vi "login3.vi"() -> ()   [LabVIEW 2023]
panel:
  in  "Tab Control":enum32{"Page 1", "Page 2"}(tab)
  in  "refresh button":bool
  in  "Username":string
  in  "Password":string
  out "LED":bool
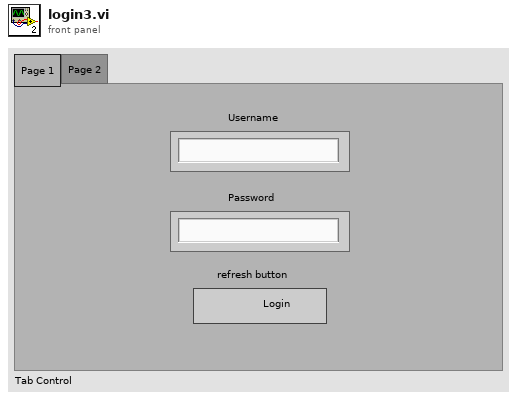
[diagram p1: front panel]
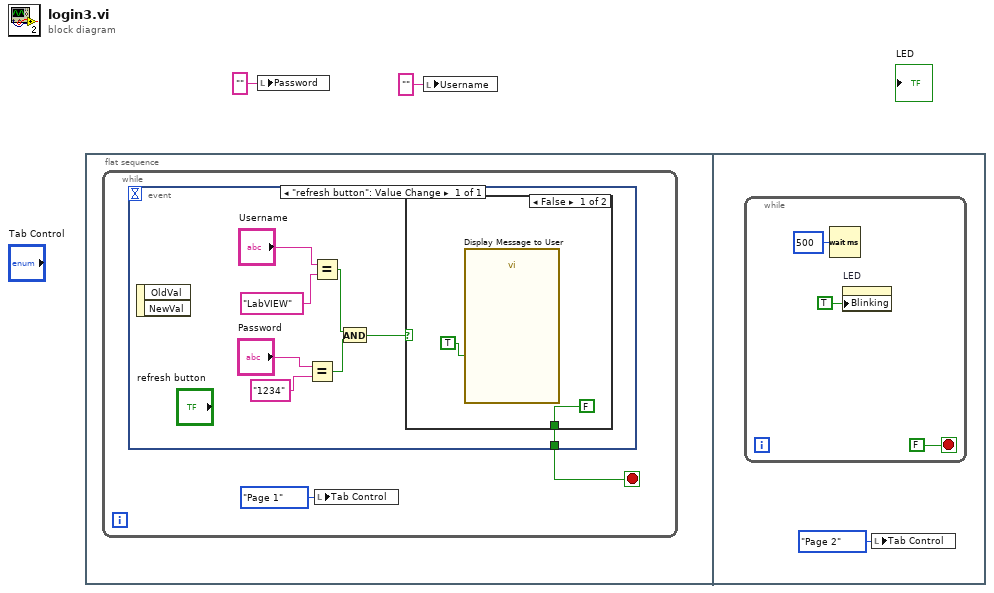
[diagram p0: block diagram]
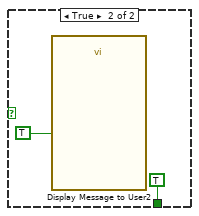
[diagram p2: hidden frame]
diagram:
  n1 = flat-sequence {
    frame #0 {
      n2 = while {
        stop <- w4 stop-if-true
        n3 = event shown="[0] \"refresh button\": Value Change" {
          selector: _ -> [_]
          dyn-events: _ -> [_]
          timeout: _ -> [_]
          tunnel: [w5] -> w4
          event "refresh button": Value Change {
            n4 = event-data() -> ()  [unwired: 1 in, 2 out]
            n5 = Equal?(x="Password", y="1234") -> (x = y?=w9:bool)
            n6 = Equal?(x="Username", y="LabVIEW") -> (x = y?=w10:bool)
            n7 = And(x=w10, y=w9) -> (x .and. y?=w8:bool)
            n8 = case shown="False" w8 {
              tunnel: [FALSE TRUE] -> w5
              frame False {
                n9 = call "Display Message to User"("Enable"=TRUE) -> ()  [unwired: 9 in, 2 out]
              }
              frame True {
                n10 = call "Display Message to User2"("Enable"=TRUE) -> ()  [unwired: 9 in, 2 out]
              }
            }
          }
        }
        n11 = local write "Tab Control"(enum32{"Page 1", "Page 2"}."Page 1" ("Tab Control")) -> ()
      }
    }
    frame #1 {
      n12 = while {
        stop <- FALSE stop-if-true
        n13 = Wait (ms)(milliseconds to wait=u32 500) -> ()  [unwired: 1 out]
        n14 = property on="LED" class="Bool (strict)"("Blinking"=TRUE) -> ()  [unwired: 2 in, 2 out]
      }
      n15 = local write "Tab Control"(enum32{"Page 1", "Page 2"}."Page 2" ("Tab Control")) -> ()
    }
  }
  n16 = local write "Password"("" ("Password")) -> ()
  n17 = local write "Username"("" ("Username")) -> ()
